vi "Folder - Create Year-Month.vi"(8 "error in (no error)":errorcluster, 11 "Folder Name":path) -> (0 "error out":errorcluster, 3 "Folder with Year\\Month":path)   [LabVIEW 2013]
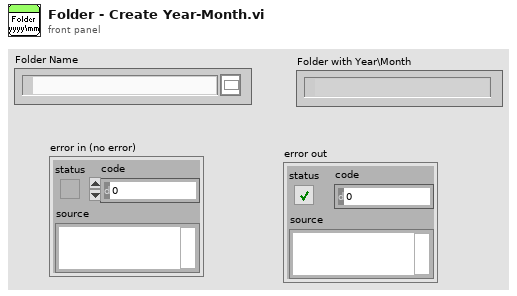
[diagram p1: front panel]
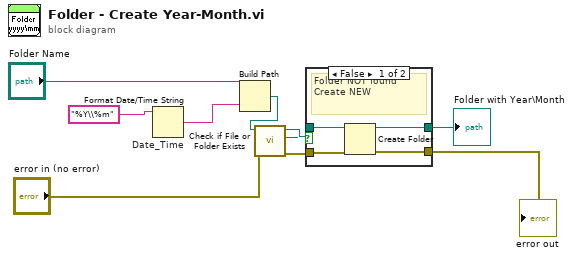
[diagram p0: block diagram]
diagram:
  n1 = Format Date/Time String "Date_Time"(time format string (%c)="%Y\\%m") -> (date/time string=w9:string)  [unwired: 2 in]
  n2 = Build Path(base path="Folder Name", name or relative path=w9) -> (appended path=w5:path)
  n3 = call <vilib>:"Check if File or Folder Exists.vi"("error in (no error)"="error in (no error)", "path"=w5) -> ("error out"=w8:errorcluster, "file or folder exists?"=w6:bool, "dup path"=w7:path)  [unwired: 7 in]
  n4 = case shown="False" w6 {
    tunnel: w7 -> [w14 w16]
    tunnel: [w13 w16] -> w3
    tunnel: [w12 w15] -> w1
    tunnel: w8 -> [w11 w15]
    frame False {
      # "Folder NOT found\nCreate NEW"
      n5 = Create Folder(path (use dialog)=w14, error in=w11) -> (created path=w13:path, error out=w12:errorcluster)  [unwired: 1 in, 1 out]
    }
    frame True {
      # "Folder Found"
    }
  }
  "Folder with Year\\Month" <- w3
  "error out" <- w1
